vi "addIDs.vi"(8 "error in (no error)":errorcluster, 10 "new IDs":u32[](array[numeric]), 11 "Structure in":refnum<class "Structure.lvclass">) -> (0 "error out":errorcluster, 3 "Structure out":refnum<class "Structure.lvclass">)   [LabVIEW 2009, in "Structure.lvclass"]
doc: "Adds new node IDs to the ID list."
uses:
  Structure.lvclass
  Structure.lvclass/Structure.ctl
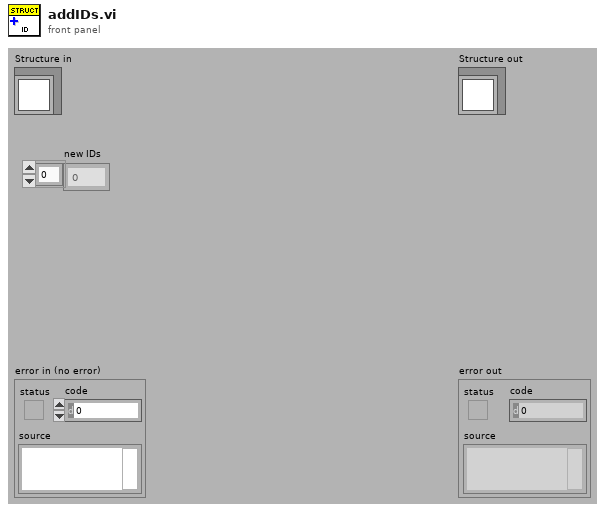
[diagram p1: front panel]
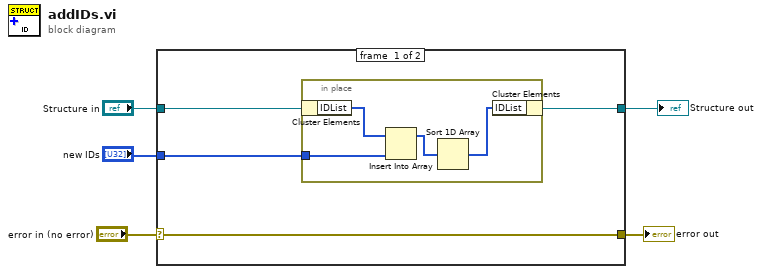
[diagram p0: block diagram]
diagram:
  n1 = case shown="No Error" "error in (no error)" {
    selector: "error in (no error)" -> [w9 w15]
    tunnel: [w9 w15] -> w4
    tunnel: [w6 w14] -> w2
    tunnel: "Structure in" -> [w8 w14]
    tunnel: "new IDs" -> [w7 _]
    frame #0 {
      n2 = in-place {
        in-place-border: w7 -> [w12]
        n3 = in-place-cluster #1(w8) -> ("IDList"=w13:u32[])
        n4 = Insert Into Array(array=w13, new element=w12) -> (w11:u32[])  [unwired: 1 in]
        n5 = Sort 1D Array(array=w11) -> (sorted array=w10:u32[])
        n6 = in-place-cluster #1("IDList"=w10) -> (w6:refnum<class "Structure.lvclass">)
      }
    }
    frame #1 {
    }
  }
  "error out" <- w4
  "Structure out" <- w2
